vi "Initialize Moxom Differential Steering.vi"(8 "error in (no error)":errorcluster) -> (0 "error out":errorcluster, 3 "differential steering frame out":refnum<class "NI_Robotics_Differential Steering Frame.lvclass">)   [LabVIEW 2011]
uses:
  <vilib>/robotics/Steering/Differential Steering Frame/Differential Wheel Group.ctl
  <vilib>/robotics/Steering/Fixed Wheel/NI_Robotics_Fixed Wheel.lvclass
  <vilib>/robotics/Steering/Differential Steering Frame/NI_Robotics_Differential Steering Frame.lvclass
  <vilib>/robotics/Actuation/Motor Communication Ref/NI_Robotics_Motor Communication Ref.lvclass
  <vilib>/robotics/Steering/Wheel/Rotation Direction.ctl
  <vilib>/robotics/Steering/Wheel/Wheel Parameters.ctl
  Robot Parameters/Robot Parameters.vi
  <vilib>/robotics/Steering/Fixed Wheel/Create Fixed Wheel.vi
  <vilib>/robotics/Steering/Differential Steering Frame/Create Differential Steering Frame.vi
  <vilib>/robotics/Steering/Wheel/NI_Robotics_Wheel.lvclass
  <vilib>/robotics/Steering/Steering Frame/NI_Robotics_Steering Frame.lvclass
panel:
  in  "wheels":T1
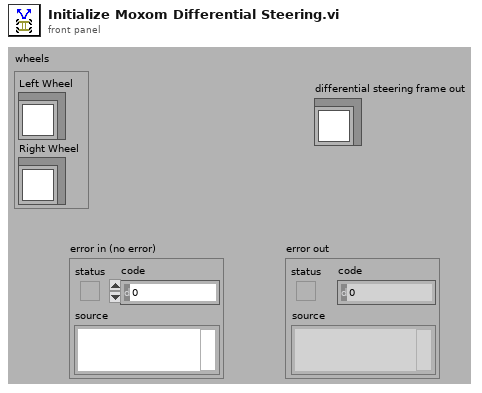
[diagram p1: front panel]
types:
  T1 = typedef "NI_Robotics_Differential Steering Frame.lvclass/Differential Wheel Group.ctl" = cluster{"Left Wheel":refnum<class "NI_Robotics_Fixed Wheel.lvclass">, "Right Wheel":refnum<class "NI_Robotics_Fixed Wheel.lvclass">}
  T2 = typedef "NI_Robotics_Wheel.lvclass/Rotation Direction.ctl" = enum16{"Clockwise", "Counterclockwise"}
  T3 = typedef "NI_Robotics_Wheel.lvclass/Wheel Parameters.ctl" = cluster{"wheel radius":dbl, "gear ratio":dbl, "forward rotation direction":T2}
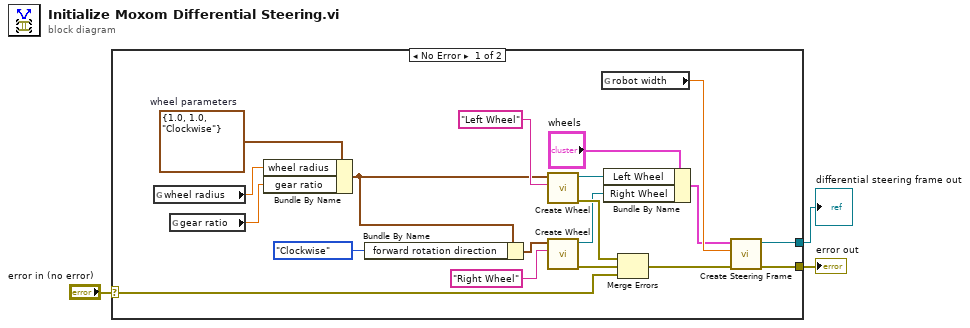
[diagram p0: block diagram]
diagram:
  n1 = case shown="No Error" "error in (no error)" {
    selector: "error in (no error)" -> [w10 w23]
    tunnel: [w21 _] -> w1
    tunnel: [w20 w23] -> w3
    frame No Error {
      w22 = T3 {"wheel radius"=1.0, "gear ratio"=1.0, "forward rotation direction"=enum."Clockwise"}  # wheel parameters
      n2 = global read "Robot Parameters.vi" "wheel radius"() -> (w18:dbl)
      n3 = global read "Robot Parameters.vi" "gear ratio"() -> (w19:dbl)
      n4 = Bundle By Name(cluster=w22, "wheel radius"=w18, "gear ratio"=w19) -> (w6:T3)
      n5 = Bundle By Name(cluster=w6, "forward rotation direction"=Rotation_Direction."Clockwise") -> (w5:T3)
      n6 = call-poly <vilib>:"Create Wheel.vi"("wheel name"="Left Wheel" ("motor name (unnamed)"), "wheel parameters"=w6) -> ("error out"=w12:errorcluster, "fixed wheel out"=w8:refnum<class "NI_Robotics_Fixed Wheel.lvclass">)  [unwired: 8 in]
      n7 = call-poly <vilib>:"Create Wheel.vi"("wheel name"="Right Wheel" ("motor name (unnamed)"), "wheel parameters"=w5) -> ("error out"=w11:errorcluster, "fixed wheel out"=w7:refnum<class "NI_Robotics_Fixed Wheel.lvclass">)  [unwired: 8 in]
      n8 = global read "Robot Parameters.vi" "robot width"() -> (w17:dbl)
      n9 = Bundle By Name(cluster="wheels", "Left Wheel"=w8, "Right Wheel"=w7) -> (w13:T1)
      n10 = Merge Errors(w12, w11, w10) -> (w9:errorcluster)
      n11 = call-poly <vilib>:"Create Steering Frame.vi"("error in (no error)"=w9, "wheel separation"=w17, "wheels"=w13) -> ("error out"=w20:errorcluster, "differential steering frame out"=w21:refnum<class "NI_Robotics_Differential Steering Frame.lvclass">)  [unwired: 7 in]
    }
    frame Error {
    }
  }
  "error out" <- w3
  "differential steering frame out" <- w1
